vi "Write Scope Characteristics.vi"(8 "error in (no error)":errorcluster, 11 "PXIe5105 in":refnum<class "PXIe5105.lvclass">) -> (0 "error out":errorcluster, 3 "PXIe5105 out":refnum<class "PXIe5105.lvclass">)   [LabVIEW 2018, in "PXIe5105.lvlib" / "PXIe5105.lvclass"]
uses:
  PXIe5105.lvclass
  PXIe5105.lvclass/PXIe5105.ctl
  <instrlib>/niScope/Controls/niScope timestamp type.ctl
  <instrlib>/niScope/Controls/niScope vertical coupling.ctl
  PPLs/Oscilloscope/Parent/Oscilloscope.lvlibp/Oscilloscope.lvclass
  PPLs/Configuration/Configuration.lvlibp/Configuration.lvclass
  C:/Projects/LabVIEW/PPLs/Oscilloscope/Parent/Oscilloscope.lvlibp/Oscilloscope.lvclass
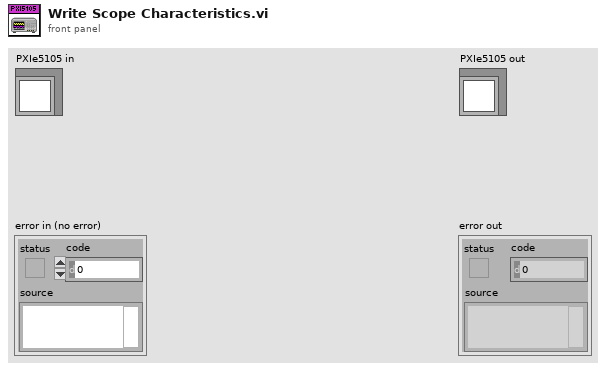
[diagram p1: front panel]
types:
  T1 = typedef "niScope timestamp type.ctl" = i32
  T2 = typedef "niScope vertical coupling.ctl" = i32
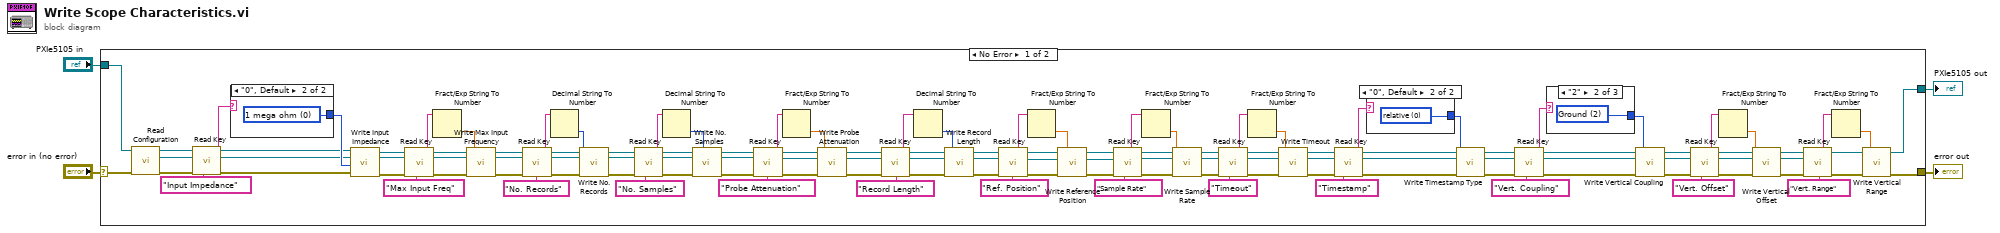
[diagram p0: block diagram]
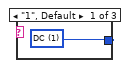
[diagram p2: hidden frame]
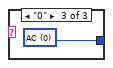
[diagram p3: hidden frame]
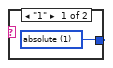
[diagram p4: hidden frame]
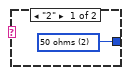
[diagram p5: hidden frame]
diagram:
  n1 = case shown="No Error" "error in (no error)" {
    selector: "error in (no error)" -> [w85 w108]
    tunnel: [w91 w108] -> w3
    tunnel: [w90 w107] -> w1
    tunnel: "PXIe5105 in" -> [w86 w107]
    frame No Error {
      n2 = call "Read Configuration.vi"("error in (no error)"=w85, "Oscilloscope in"=w86) -> ("error out"=w87:errorcluster, "Configuration"=w88:refnum<class "Configuration.lvclass">, "Oscilloscope out"=w81:refnum<class "PXIe5105.lvclass">)  [unwired: 7 in]
      n3 = call "Read Key.vi"("Key:"="Input Impedance", "error in"=w87, "Configuration in"=w88) -> ("error out"=w82:errorcluster, "Value"=w84:string, "Configuration out"=w80:refnum<class "Configuration.lvclass">)  [unwired: 6 in]
      n4 = case shown="\"0\", Default" w84 {
        tunnel: [w105 w106] -> w83
        frame "2" {
          w105 = u32 2 items=["1 mega ohm"=0, "50 ohms"=2] ("Input Impedance")
        }
        frame "0", Default {
          w106 = u32 0 items=["1 mega ohm"=0, "50 ohms"=2] ("Input Impedance")
        }
      }
      n5 = call "Write Input Impedance.vi"("error in (no error)"=w82, "Input Impedance"=w83, "PXIe5105 in"=w81) -> ("error out"=w79:errorcluster, "PXIe5105 out"=w99:refnum<class "PXIe5105.lvclass">)  [unwired: 7 in]
      n6 = call "Read Key.vi"("Key:"="Max Input Freq", "error in"=w79, "Configuration in"=w80) -> ("error out"=w75:errorcluster, "Value"=w77:string, "Configuration out"=w68:refnum<class "Configuration.lvclass">)  [unwired: 6 in]
      n7 = Fract/Exp String To Number(string=w77) -> (number=w76:dbl)  [unwired: 3 in, 1 out]
      n8 = call "Write Max Input Frequency.vi"("error in (no error)"=w75, "Max Input Frequency"=w76, "PXIe5105 in"=w99) -> ("error out"=w72:errorcluster, "PXIe5105 out"=w69:refnum<class "PXIe5105.lvclass">)  [unwired: 7 in]
      n9 = call "Read Key.vi"("Key:"="No. Records", "error in"=w72, "Configuration in"=w68) -> ("error out"=w71:errorcluster, "Value"=w74:string, "Configuration out"=w65:refnum<class "Configuration.lvclass">)  [unwired: 6 in]
      n10 = Decimal String To Number(string=w74) -> (number=w70:i32)  [unwired: 2 in, 1 out]
      n11 = call "Write No. Records.vi"("error in (no error)"=w71, "No. Records"=w70, "PXIe5105 in"=w69) -> ("error out"=w67:errorcluster, "PXIe5105 out"=w66:refnum<class "PXIe5105.lvclass">)  [unwired: 7 in]
      n12 = call "Read Key.vi"("Key:"="No. Samples", "error in"=w67, "Configuration in"=w65) -> ("error out"=w62:errorcluster, "Value"=w63:string, "Configuration out"=w59:refnum<class "Configuration.lvclass">)  [unwired: 6 in]
      n13 = Decimal String To Number(string=w63) -> (number=w61:i32)  [unwired: 2 in, 1 out]
      n14 = call "Write No. Samples.vi"("error in (no error)"=w62, "No. Samples"=w61, "PXIe5105 in"=w66) -> ("error out"=w58:errorcluster, "PXIe5105 out"=w60:refnum<class "PXIe5105.lvclass">)  [unwired: 7 in]
      n15 = call "Read Key.vi"("Key:"="Probe Attenuation", "error in"=w58, "Configuration in"=w59) -> ("error out"=w54:errorcluster, "Value"=w56:string, "Configuration out"=w50:refnum<class "Configuration.lvclass">)  [unwired: 6 in]
      n16 = Fract/Exp String To Number(string=w56) -> (number=w55:dbl)  [unwired: 3 in, 1 out]
      n17 = call "Write Probe Attenuation.vi"("error in (no error)"=w54, "Probe Attenuation"=w55, "PXIe5105 in"=w60) -> ("error out"=w53:errorcluster, "PXIe5105 out"=w98:refnum<class "PXIe5105.lvclass">)  [unwired: 7 in]
      n18 = call "Read Key.vi"("Key:"="Record Length", "error in"=w53, "Configuration in"=w50) -> ("error out"=w52:errorcluster, "Value"=w49:string, "Configuration out"=w46:refnum<class "Configuration.lvclass">)  [unwired: 6 in]
      n19 = Decimal String To Number(string=w49) -> (number=w48:i32)  [unwired: 2 in, 1 out]
      n20 = call "Write Record Length.vi"("error in (no error)"=w52, "Record Length"=w48, "PXIe5105 in"=w98) -> ("error out"=w42:errorcluster, "PXIe5105 out"=w47:refnum<class "PXIe5105.lvclass">)  [unwired: 7 in]
      n21 = call "Read Key.vi"("Key:"="Ref. Position", "error in"=w42, "Configuration in"=w46) -> ("error out"=w41:errorcluster, "Value"=w44:string, "Configuration out"=w40:refnum<class "Configuration.lvclass">)  [unwired: 6 in]
      n22 = Fract/Exp String To Number(string=w44) -> (number=w43:dbl)  [unwired: 3 in, 1 out]
      n23 = call "Write Reference Position.vi"("error in (no error)"=w41, "Reference Position"=w43, "PXIe5105 in"=w47) -> ("error out"=w39:errorcluster, "PXIe5105 out"=w97:refnum<class "PXIe5105.lvclass">)  [unwired: 7 in]
      n24 = call "Read Key.vi"("Key:"="Sample Rate", "error in"=w39, "Configuration in"=w40) -> ("error out"=w37:errorcluster, "Value"=w36:string, "Configuration out"=w33:refnum<class "Configuration.lvclass">)  [unwired: 6 in]
      n25 = Fract/Exp String To Number(string=w36) -> (number=w35:dbl)  [unwired: 3 in, 1 out]
      n26 = call "Write Sample Rate.vi"("error in (no error)"=w37, "Sample Rate"=w35, "PXIe5105 in"=w97) -> ("error out"=w32:errorcluster, "PXIe5105 out"=w96:refnum<class "PXIe5105.lvclass">)  [unwired: 7 in]
      n27 = call "Read Key.vi"("Key:"="Timeout", "error in"=w32, "Configuration in"=w33) -> ("error out"=w31:errorcluster, "Value"=w30:string, "Configuration out"=w26:refnum<class "Configuration.lvclass">)  [unwired: 6 in]
      n28 = Fract/Exp String To Number(string=w30) -> (number=w29:dbl)  [unwired: 3 in, 1 out]
      n29 = call "Write Timeout.vi"("error in (no error)"=w31, "Timeout"=w29, "PXIe5105 in"=w96) -> ("error out"=w25:errorcluster, "PXIe5105 out"=w95:refnum<class "PXIe5105.lvclass">)  [unwired: 7 in]
      n30 = call "Read Key.vi"("Key:"="Timestamp", "error in"=w25, "Configuration in"=w26) -> ("error out"=w24:errorcluster, "Value"=w28:string, "Configuration out"=w20:refnum<class "Configuration.lvclass">)  [unwired: 6 in]
      n31 = case shown="\"0\", Default" w28 {
        tunnel: [w103 w104] -> w23
        frame "1" {
          w103 = T1 1 items=["relative", "absolute"] ("Tmestamp Type")
        }
        frame "0", Default {
          w104 = T1 0 items=["relative", "absolute"] ("Tmestamp Type")
        }
      }
      n32 = call "Write Timestamp Type.vi"("error in (no error)"=w24, "timestamp type"=w23, "PXIe5105 in"=w95) -> ("error out"=w19:errorcluster, "PXIe5105 out"=w94:refnum<class "PXIe5105.lvclass">)  [unwired: 7 in]
      n33 = call "Read Key.vi"("Key:"="Vert. Coupling", "error in"=w19, "Configuration in"=w20) -> ("error out"=w18:errorcluster, "Value"=w22:string, "Configuration out"=w13:refnum<class "Configuration.lvclass">)  [unwired: 6 in]
      n34 = case shown="\"2\"" w22 {
        tunnel: [w100 w101 w102] -> w17
        frame "1", Default {
          w100 = T2 1 items=["AC", "DC", "Ground"] ("vertical coupling")
        }
        frame "2" {
          w101 = T2 2 items=["AC", "DC", "Ground"] ("vertical coupling")
        }
        frame "0" {
          w102 = T2 0 items=["AC", "DC", "Ground"] ("vertical coupling")
        }
      }
      n35 = call "Write Vertical Coupling.vi"("error in (no error)"=w18, "vertical coupling"=w17, "PXIe5105 in"=w94) -> ("error out"=w14:errorcluster, "PXIe5105 out"=w93:refnum<class "PXIe5105.lvclass">)  [unwired: 7 in]
      n36 = call "Read Key.vi"("Key:"="Vert. Offset", "error in"=w14, "Configuration in"=w13) -> ("error out"=w12:errorcluster, "Value"=w16:string, "Configuration out"=w8:refnum<class "Configuration.lvclass">)  [unwired: 6 in]
      n37 = Fract/Exp String To Number(string=w16) -> (number=w11:dbl)  [unwired: 3 in, 1 out]
      n38 = call "Write Vertical Offset.vi"("error in (no error)"=w12, "Vertical Offset"=w11, "PXIe5105 in"=w93) -> ("error out"=w9:errorcluster, "PXIe5105 out"=w92:refnum<class "PXIe5105.lvclass">)  [unwired: 7 in]
      n39 = call "Read Key.vi"("Key:"="Vert. Range", "error in"=w9, "Configuration in"=w8) -> ("error out"=w5:errorcluster, "Value"=w10:string)  [unwired: 6 in, 1 out]
      n40 = Fract/Exp String To Number(string=w10) -> (number=w6:dbl)  [unwired: 3 in, 1 out]
      n41 = call "Write Vertical Range.vi"("error in (no error)"=w5, "Vertical Range"=w6, "PXIe5105 in"=w92) -> ("error out"=w91:errorcluster, "PXIe5105 out"=w90:refnum<class "PXIe5105.lvclass">)  [unwired: 7 in]
    }
    frame Error {
    }
  }
  "error out" <- w3
  "PXIe5105 out" <- w1
